vi "Override Error.vi"(10 "Error":errorcluster, 11 "jettl Actor in":refnum<class "jettl Actor.lvclass">) -> (3 "jettl Actor out":refnum<class "jettl Actor.lvclass">)   [LabVIEW 2021, in "jettl.lvlib" / "Temporary Actor.lvlib" / "jettl Actor.lvclass"]
uses:
  jettl Actor.lvclass
  jettl Actor.lvclass/jettl Actor.ctl
  State.ctl
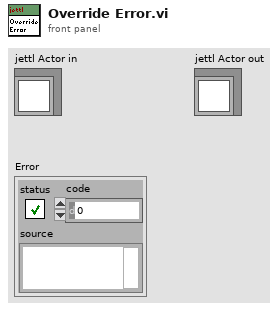
[diagram p1: front panel]
types:
  T1 = typedef "jettl.lvlib/Temporary Actor.lvlib/jettl Actor.lvclass/State.ctl" = enum16{"Nominal", "Teardown", "Error"}
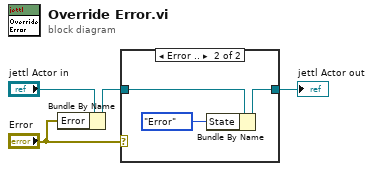
[diagram p0: block diagram]
diagram:
  n1 = Bundle By Name(cluster="jettl Actor in", "Error"="Error") -> (w3:refnum<class "jettl Actor.lvclass">)
  n2 = case shown="Error .." "Error" {
    tunnel: [w5 w7] -> w2
    tunnel: w3 -> [w5 w8]
    frame No Error {
    }
    frame Error {
      n3 = Bundle By Name(cluster=w8, "State"=State."Error") -> (w7:refnum<class "jettl Actor.lvclass">)
    }
  }
  "jettl Actor out" <- w2
